vi "Multi Channel Stream - Many Channels.vi"() -> ()   [LabVIEW 2020]
uses:
  Stream/Stream.lvclass
  <vilib>/Utility/config.llb/NI_LVConfig.lvlib
  <vilib>/Utility/config.llb/Read Key (String).vi
panel:
  in  "Stop":bool
  in  "Number of channels":i32=10 min=1 max=200
  out "appended path":path
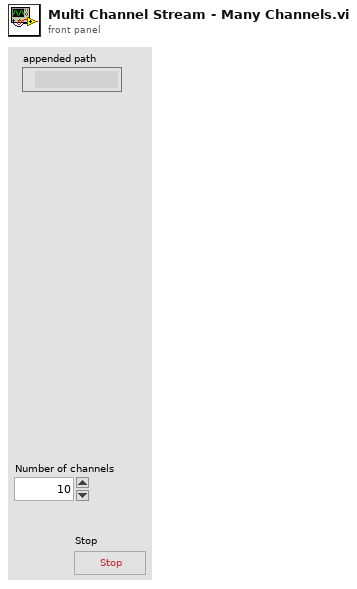
[diagram p1: front panel]
types:
  T1 = typedef "NI_LVConfig.lvlib/Config Data RefNum.ctl" = refnum<k1>
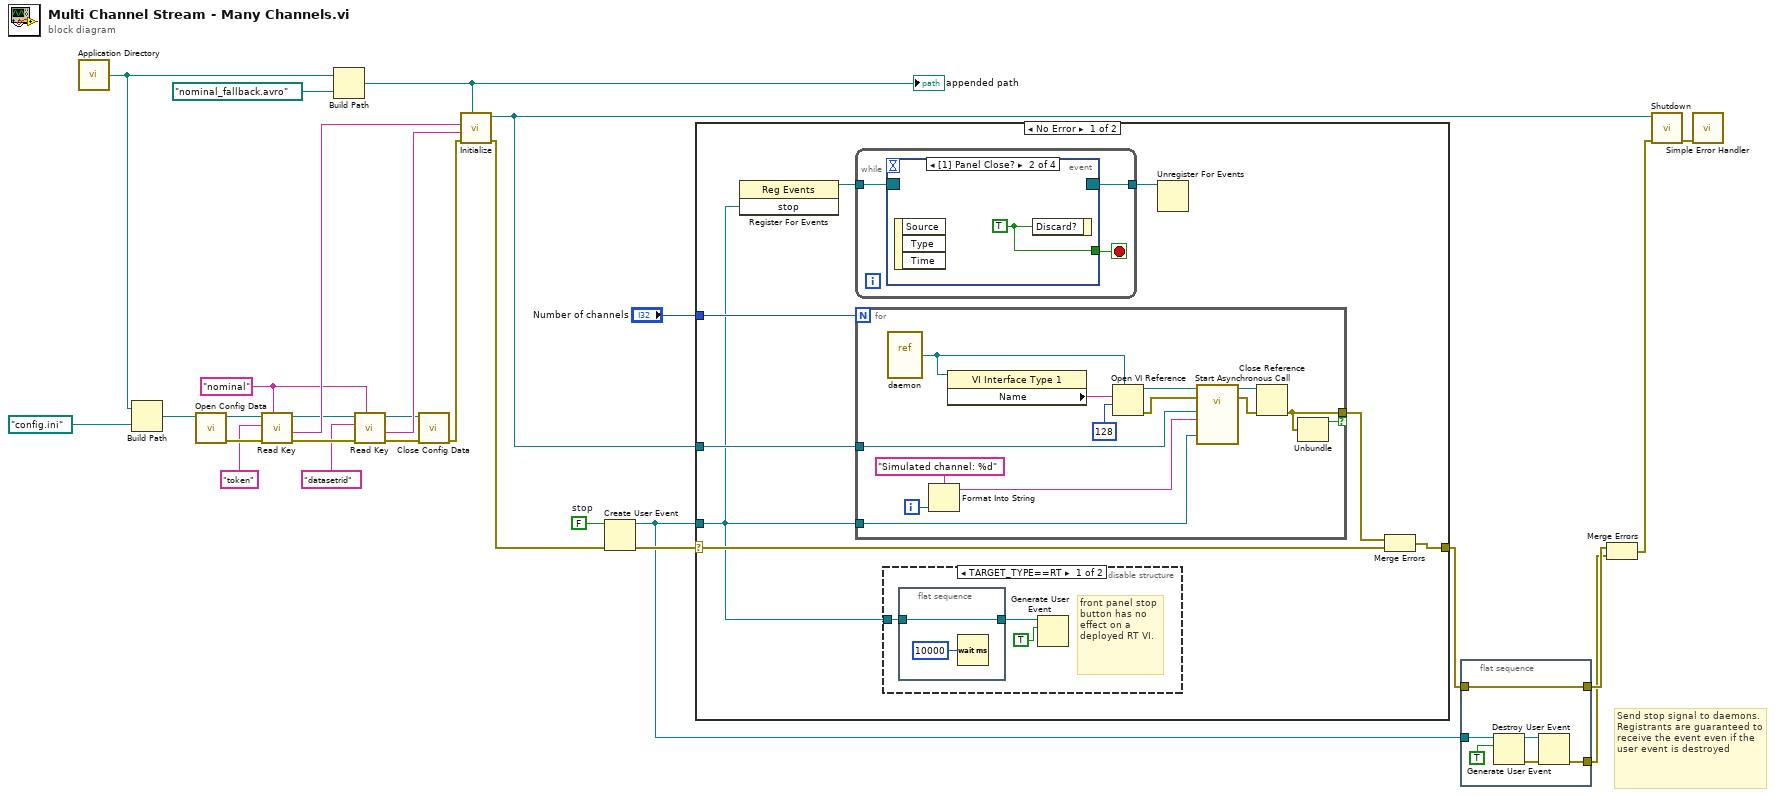
[diagram p0: block diagram]
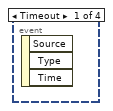
[diagram p3: hidden frame]
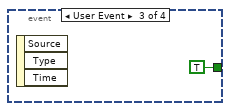
[diagram p4: hidden frame]
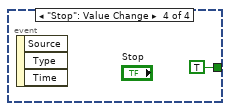
[diagram p5: hidden frame]
diagram:
  w1 = "nominal" ("section")
  w23 = FALSE  # stop
  # "Send stop signal to daemons.\nRegistrants are guaranteed to receive the event even if the user event is destroyed"
  n1 = call <vilib>:"Application Directory.vi"() -> ("Application Directory"=w24:path)
  n2 = Build Path(base path=w24, name or relative path=path "config.ini") -> (appended path=w10:path)
  n3 = call <vilib>:"Open Config Data.vi"("configuration file path"=w10) -> ("error out"=w4:errorcluster, "refnum"=w9:T1)  [unwired: 8 in, 1 out]
  n4 = call-poly <vilib>:"Read Key.vi"("section"=w1, "error in (no error)"=w4, "key"="token", "refnum"=w9) -> ("error out"=w5:errorcluster, "value"=w26:string, "refnum out"=w8:T1)  [unwired: 4 in, 1 out]
  n5 = Build Path(base path=w24, name or relative path=path "nominal_fallback.avro") -> (appended path=w27:path)
  "appended path" <- w27
  n6 = call-poly <vilib>:"Read Key.vi"("section"=w1, "error in (no error)"=w5, "key"="datasetrid", "refnum"=w8) -> ("error out"=w6:errorcluster, "value"=w25:string, "refnum out"=w7:T1)  [unwired: 4 in, 1 out]
  n7 = call <vilib>:"Close Config Data.vi"("error in (no error)"=w6, "refnum"=w7) -> ("error out"=w18:errorcluster)  [unwired: 8 in, 1 out]
  n8 = call "Initialize.vi"("Fallback File Path"=w27, "error in (no error)"=w18, "Dataset RID"=w25, "Token"=w26) -> ("error out"=w20:errorcluster, "Nominal Streaming out"=w21:refnum<class "Stream.lvclass">)  [unwired: 6 in]
  n9 = Create User Event(user event datatype=w23, error in=w20) -> (user event=w12:refnum<user-event>, error out=w19:errorcluster)
  n10 = case shown="No Error" w19 {
    selector: w19 -> [w33 w62]
    tunnel: "Number of channels" -> [w36 _]
    tunnel: w21 -> [w35 _]
    tunnel: w12 -> [w30 _]
    tunnel: [w32 w62] -> w17
    frame No Error {
      n11 = register-events(w30) -> (reference out=w31:refnum<event-registration>)  [unwired: 2 in, 1 out]
      n12 = while {
        tunnel: w31 -> [w43]
        tunnel: [w42] -> w29
        stop <- w44 stop-if-true
        n13 = event shown="[1] Panel Close?" {
          selector: w43 -> [_ _ _ _]
          dyn-events: [_ _ _ _] -> w42
          timeout: _ -> [_ _ _ _]
          tunnel: [_ w45 TRUE ("Discard?") TRUE ("Discard?")] -> w44
          event Timeout {
            n14 = event-data() -> ()  [unwired: 1 in, 3 out]
          }
          event Panel Close? {
            w45 = TRUE ("Discard?")
            n15 = event-data() -> ()  [unwired: 1 in, 3 out]
            n16 = event-data("Discard?"=w45) -> ()  [unwired: 1 in, 1 out]
          }
          event User Event {
            n17 = event-data() -> ()  [unwired: 1 in, 3 out]
          }
          event "Stop": Value Change {
            n18 = event-data() -> ()  [unwired: 1 in, 3 out]
          }
        }
      }
      n19 = for {
        N: w36 -> [_]
        tunnel: w30 -> [w57]
        tunnel: w35 -> [w55]
        tunnel: [w49] -> w34 if=w48
        i -> [w53]
        n20 = vi-ref "daemon.vi"() -> (w56:refnum<vi>)
        n21 = Format Into String(format string="Simulated channel: %d", w53) -> (resulting string=w52:string)  [unwired: 2 in, 1 out]
        n22 = property class="VI Interface Type 1"(reference=w56) -> ("Name"=w59:string)  [unwired: 1 in, 2 out]
        n23 = Open VI Reference(type specifier VI Refnum (for type only)=w56, vi path=w59, options=128) -> (vi reference=w60:refnum<vi>, error out=w61:errorcluster)  [unwired: 3 in]
        n24 = call-by-ref "Start Asynchronous Call"(reference=w60, error in=w61, "stop"=w57, "Channel Name"=w52, "Nominal Streaming in"=w55) -> (reference out=w51:refnum<vi>, error out=w50:errorcluster)  [unwired: 9 in]
        n25 = Close Reference(reference=w51, error in (no error)=w50) -> (error out=w49:errorcluster)
        n26 = Unbundle(w49) -> ("status"=w48:bool)  [unwired: 2 out]
      }
      n27 = disable-structure shown="TARGET_TYPE==RT" {
        disable-tunnel: w30 -> [w38 _]
        frame condition #0 (active) {
          # "front panel stop button has no effect on a deployed RT VI."
          n28 = flat-sequence {
            tunnel: w38 -> [w40]
            tunnel: [w40] -> w37
            frame #0 {
              n29 = Wait (ms)(milliseconds to wait=u32 10000) -> ()  [unwired: 1 out]
            }
          }
          n30 = Generate User Event(user event=w37, event data cluster=TRUE ("event data")) -> ()  [unwired: 2 in, 2 out]
        }
        frame condition #1 {
        }
      }
      n31 = Unregister For Events(event registration refnum=w29) -> ()  [unwired: 1 in, 1 out]
      n32 = Merge Errors(w34, w33) -> (w32:errorcluster)
    }
    frame Error {
    }
  }
  n33 = flat-sequence {
    tunnel: [w66] -> w15
    tunnel: w12 -> [w64]
    tunnel: [w63] -> w16
    tunnel: w17 -> [w63]
    frame #0 {
      n34 = Generate User Event(user event=w64, event data cluster=TRUE ("event data")) -> (user event out=w68:refnum<user-event>, error out=w65:errorcluster)  [unwired: 2 in]
      n35 = Destroy User Event(user event=w68, error in=w65) -> (error out=w66:errorcluster)
    }
  }
  n36 = Merge Errors(w16, w15) -> (w14:errorcluster)
  n37 = call "Shutdown.vi"("error in (no error)"=w14, "Nominal Streaming in"=w21) -> ("error out"=w13:errorcluster)  [unwired: 8 in, 1 out]
  n38 = call <vilib>:"Simple Error Handler.vi"("error in (no error)"=w13) -> ()  [unwired: 4 in, 5 out]
